vi "Write Trigger.vi"(8 "error in (no error)":errorcluster, 10 "Trigger":T1, 11 "SpecAnBase in":refnum<class "SpecAnBase.lvclass">) -> (0 "error out":errorcluster, 3 "SpecAnBase out":refnum<class "SpecAnBase.lvclass">)   [LabVIEW 2018, in "SpecAnPlugins.lvlib" / "SpecAnBase.lvclass"]
uses:
  SpecAnBase.lvclass
  SpecAnBase.lvclass/SpecAnBase.ctl
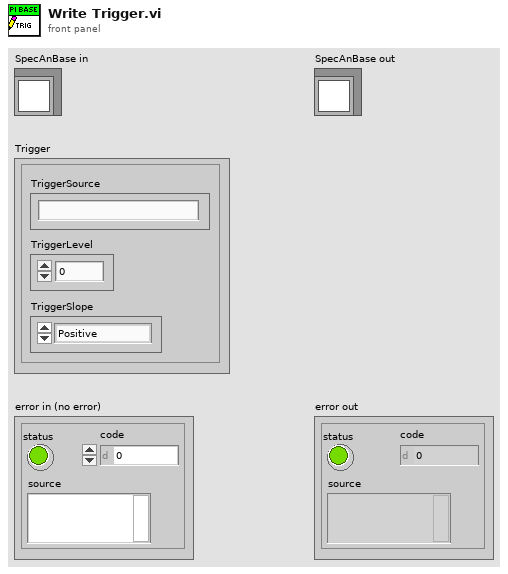
[diagram p1: front panel]
types:
  T1 = cluster{"TriggerSource":string, "TriggerLevel":dbl, "TriggerSlope":enum16{"Positive", "Negative"}}
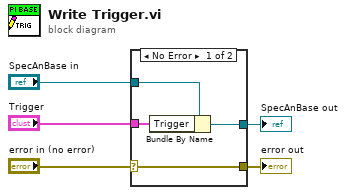
[diagram p0: block diagram]
diagram:
  n1 = case shown="No Error" "error in (no error)" {
    selector: "error in (no error)" -> [w9 w10]
    tunnel: [w9 w10] -> w4
    tunnel: [w7 w11] -> w2
    tunnel: "SpecAnBase in" -> [w8 w11]
    tunnel: "Trigger" -> [w6 _]
    frame No Error {
      n2 = Bundle By Name(cluster=w8, "Trigger"=w6) -> (w7:refnum<class "SpecAnBase.lvclass">)
    }
    frame Error {
    }
  }
  "error out" <- w4
  "SpecAnBase out" <- w2
